vi "SendPanicEmail.vi"(8 "ErrorIn":errorcluster, 10 "DIALNumber":string, 11 "TypeOfEmail":bool) -> (0 "ErrorOut":errorcluster)   [LabVIEW 2012]
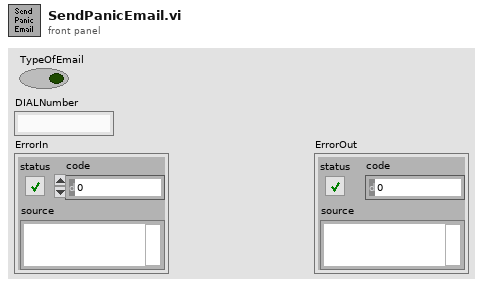
[diagram p1: front panel]
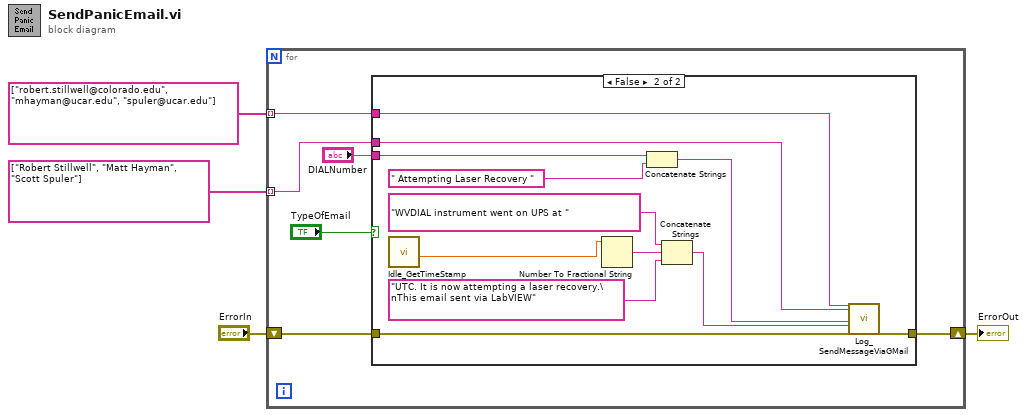
[diagram p0: block diagram]
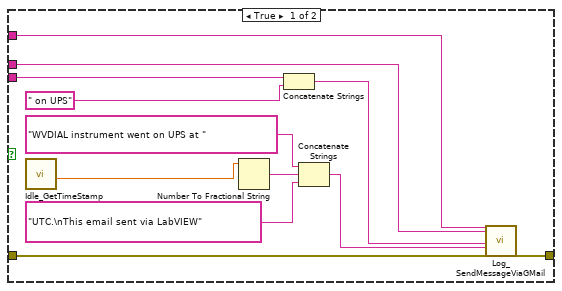
[diagram p2: hidden frame]
diagram:
  n1 = for {
    shift-right: [w9] -> w1
    shift-left: "ErrorIn" -> [w8]
    tunnel: string[] ["robert.stillwell@colorado.edu", "mhayman@ucar.edu", "spuler@ucar.edu"] -> [w7] mode=indexing
    tunnel: string[] ["Robert Stillwell", "Matt Hayman", "Scott Spuler"] -> [w6] mode=indexing
    n2 = case shown="False" "TypeOfEmail" {
      tunnel: w8 -> [w22 w34]
      tunnel: [w21 w33] -> w9
      tunnel: w7 -> [w13 w25]
      tunnel: w6 -> [w12 w24]
      tunnel: "DIALNumber" -> [w11 w23]
      frame True {
        n3 = call "Idle_GetTimeStamp.vi"() -> ("Fractional Hours"=w17:dbl)  [unwired: 11 in]
        n4 = Number To Fractional String(number=w17) -> (F-format string=w19:string)  [unwired: 3 in]
        n5 = Concatenate Strings(w11, " on UPS") -> (w14:string)
        n6 = Concatenate Strings("WVDIAL instrument went on UPS at ", w19, "UTC.\nThis email sent via LabVIEW") -> (w16:string)
        n7 = call "Log_SendMessageViaGMail.vi"("Recipient's Email Address Address"=w13, "Recipient's Name"=w12, "Subject"=w14, "Body"=w16, "Error In"=w22) -> ("Error Out"=w21:errorcluster)  [unwired: 22 in]
      }
      frame False {
        n8 = call "Idle_GetTimeStamp.vi"() -> ("Fractional Hours"=w29:dbl)  [unwired: 11 in]
        n9 = Number To Fractional String(number=w29) -> (F-format string=w31:string)  [unwired: 3 in]
        n10 = Concatenate Strings(w23, " Attempting Laser Recovery ") -> (w26:string)
        n11 = Concatenate Strings("WVDIAL instrument went on UPS at ", w31, "UTC. It is now attempting a laser recovery.\nThis email sent via LabVIEW") -> (w28:string)
        n12 = call "Log_SendMessageViaGMail.vi"("Recipient's Email Address Address"=w25, "Recipient's Name"=w24, "Subject"=w26, "Body"=w28, "Error In"=w34) -> ("Error Out"=w33:errorcluster)  [unwired: 22 in]
      }
    }
  }
  "ErrorOut" <- w1
